vi "pH V over T.vi"(2 "Temperature":dbl format="%.2f", 3 "Voltage":dbl format="%.2f") -> (0 "Temperature out":dbl format="%.2f", 1 "V/T":dbl format="%.2f")   [LabVIEW 2019]
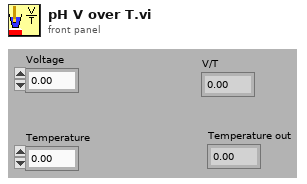
[diagram p1: front panel]
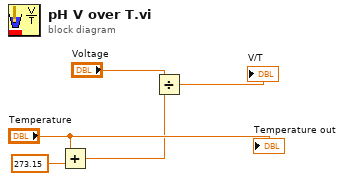
[diagram p0: block diagram]
diagram:
  n1 = Add(x="Temperature", y=273.15) -> (x+y=w3:dbl)
  n2 = Divide(x="Voltage", y=w3) -> (x/y=→"V/T":dbl)
  "Temperature out" <- "Temperature"
